vi "CODCr插入数据.vi"(0 "database":string, 1 "data":T3 {"单位" items=["ug/L", "mg/L", "ppm", "mg/m3", "cm", "ppb", "ug/m3", "%", "nmol/mol", "umol/mol", "MPN/L", "MPN/100ml", "ng/m3", "NTU", "无量纲", "ms/cm", "us/cm"]}, 5 "table":string, 7 "测量模式":T2(ring)=enum."水样测试", 9 "数据类型":enum16{"N", "M"}(ring)=enum."M", 11 "error in (no error)":errorcluster) -> (15 "error out":errorcluster)   [LabVIEW 2016, in "CODCr库.lvlib"]
uses:
  <vilib>/Utility/sysdir.llb/System Directory Type.ctl
  <vilib>/Utility/error.llb/DialogType.ctl
  <vilib>/addons/database/Auxilliary.llb/DB Tools Column Info.ctl
  <vilib>/addons/database/Auxilliary.llb/DB Tools DataTypes.ctl
  <vilib>/addons/database/Connection.llb/DB Tools Open Connec (String).vi
  <vilib>/addons/database/Connection.llb/Conn Execute.vi
  <vilib>/addons/database/Recordset.llb/Rec Destroy - Connection.vi
  <vilib>/addons/database/Recordset.llb/Rec Fetch Recordset Data (R).vi
  <vilib>/addons/database/NI_Database_API.lvlib
  WxMessage/wxpusher.lvlib
panel:
  out "data修正输出":T1
  out "data输出":T1
  out "为空？":bool
  out "recordset data":variant[][](array[variant])
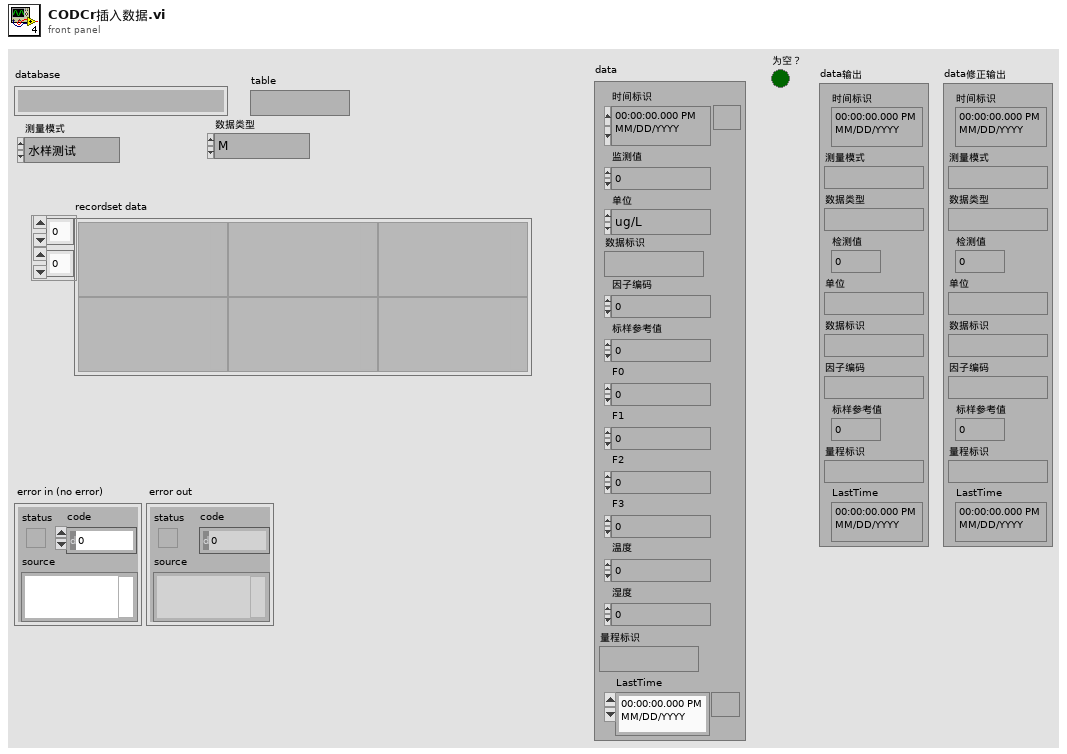
[diagram p1: front panel]
types:
  T1 = cluster{"时间标识":timestamp, "测量模式":string, "数据类型":string, "检测值":sgl, "单位":string, "数据标识":string, "因子编码":string, "标样参考值":sgl, "量程标识":string, "LastTime":timestamp}
  T2 = enum16{"空闲", "水样测试", "标样核查", "零点核查", "跨度核查", "空白测试", "平行样测试", "加标回收", "空白校准", "标样校准", "初始化（清洗）"}
  T3 = cluster{"时间标识":timestamp, "监测值":sgl, "单位":u16, "数据标识":string, "因子编码":u32, "标样参考值":sgl, "F0":sgl, "F1":sgl, "F2":sgl, "F3":sgl, "温度":sgl, "湿度":sgl, "量程标识":string, "LastTime":timestamp}
  T4 = typedef "DialogType.ctl" = u16
  T5 = typedef "System Directory Type.ctl" = i32
  T6 = typedef "NI_Database_API.lvlib/Conn ObjectReference.ctl" = refnum<k1>
  T7 = typedef "NI_Database_API.lvlib/Rec ObjectReference.ctl" = refnum<k1>
  T8 = typedef "NI_Database_API.lvlib/DB Tools Column Info.ctl" = cluster{"column name":string, "data type":T9, "size":i32, "allow null?":bool}
  T9 = typedef "NI_Database_API.lvlib/DB Tools DataTypes.ctl" = enum16{"String", "Long (I32)", "Single (SGL)", "Double (DBL)", "Date/Time", "Binary"}
  T10 = cluster{"测量量程":dbl, "测量精度":dbl, "测量间隔":dbl, "消解温度":dbl, "消解时长":dbl, "空白校准时间":timestamp, "曲线截距":dbl, "曲线斜率":dbl, "测量检出限":dbl, "测量信号值":dbl, "线性相关系数":dbl, "二次多项式系数":dbl, "标样校准时间":timestamp, "稀释倍数":dbl, "三项式系数":dbl, "空白标定系数":dbl, "量程系数":dbl, "F0/ORPA":dbl, "F1/ORPB":dbl, "F2/ORPK":dbl, "F3":dbl, "F4":dbl, "F5":dbl, "F6":dbl, "F7":dbl, "X0/滴定数":dbl, "量程":dbl}
  T11 = cluster{"切换阈值":dbl, "稳定系数":dbl, "变异系数":dbl, "enable":bool, "init":bool}
  T12 = cluster{"数值输出":dbl, "均值":dbl, "变异系数":dbl, "数据波动百分比":dbl, "随机数flag":bool}
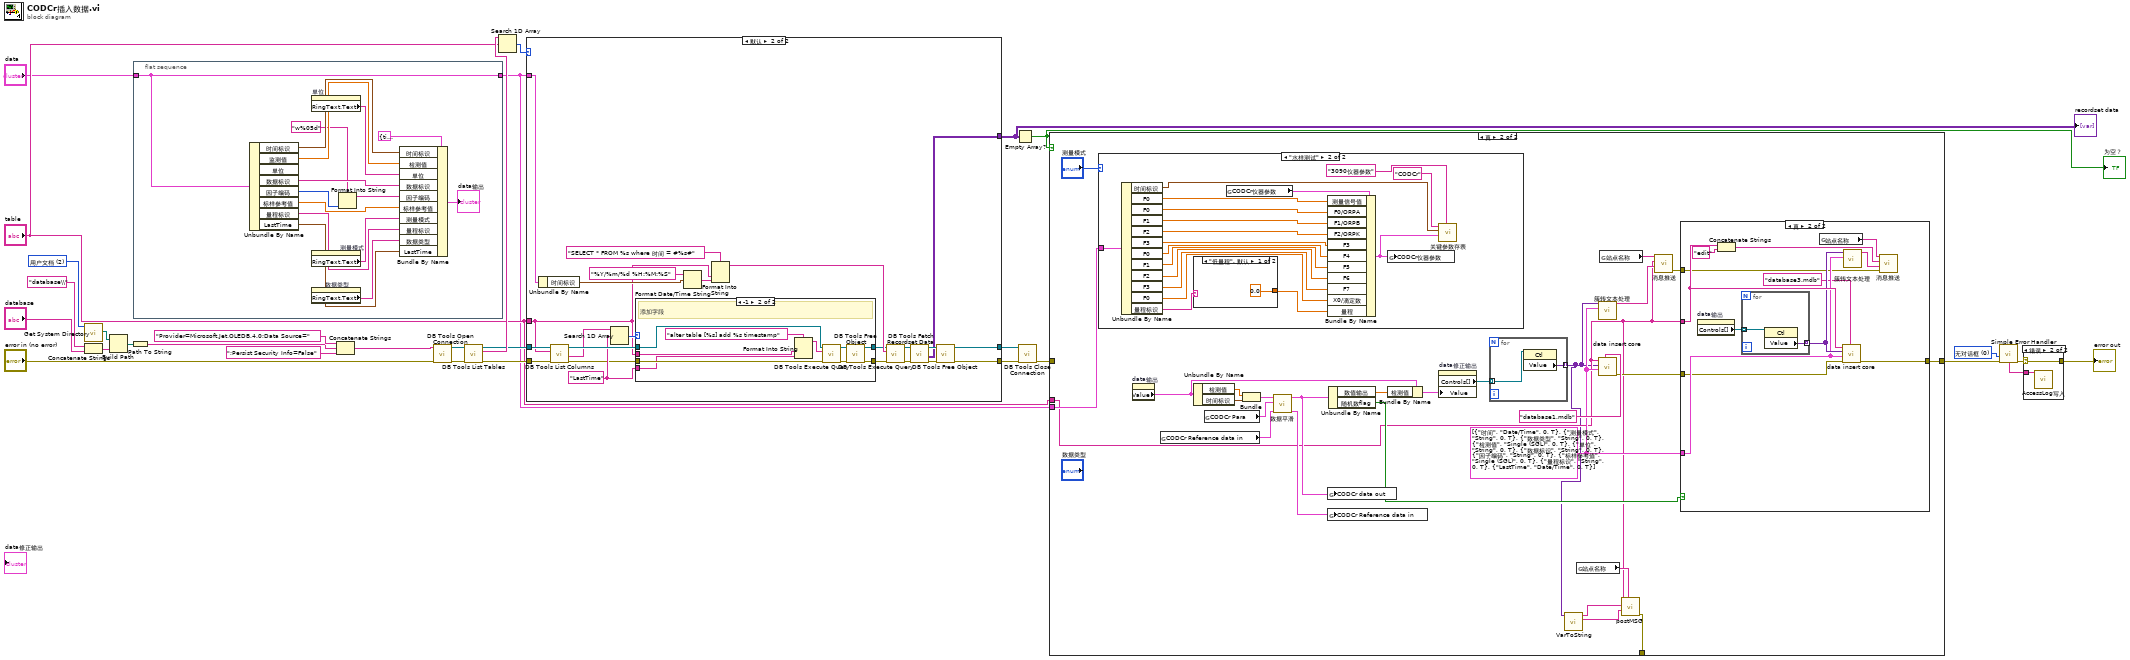
[diagram p0: block diagram]
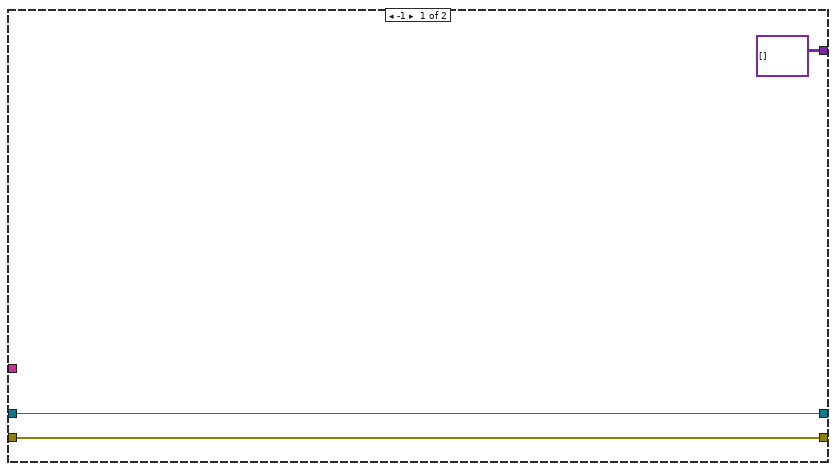
[diagram p3: hidden frame]
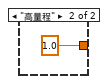
[diagram p8: hidden frame]
diagram:
  w11 = T4 0 items=["无对话框", "确定信息", "继续或停止信息", "确定信息＋警告", "继续/停止+警告"] ("type of dialog (OK msg:1)")
  w29 = T5 2 items=["用户目录"=0, "用户桌面"=1, "用户文档"=2, "用户应用程序数据"=3, "用户设置"=4, "用户临时目录"=5, "公共文档"=6, "公共应用程序数据"=7, "公共设置"=8, "公共缓存"=13, "系统核心库"=9, "系统安装库"=10, "应用程序文件"=11, "启动盘根目录"=12] ("system directory type")
  n1 = call <vilib>:"Get System Directory.vi"("system directory type"=w29) -> ("system directory"=w27:path)  [unwired: 10 in]
  n2 = Concatenate Strings("database\\" ("condition"), "database") -> (w21:string)
  n3 = Build Path(base path=w27, name or relative path=w21) -> (appended path=w26:path)
  n4 = Path To String(path=w26) -> (string=w25:string)
  n5 = flat-sequence {
    tunnel: "data" -> [w31]
    tunnel: [w31] -> w3
    frame #0 {
      n6 = Unbundle By Name(w31) -> ("时间标识"=w44:timestamp, "监测值"=w43:sgl, "数据标识"=w41:string, "因子编码"=w39:u32, "标样参考值"=w37:sgl, "量程标识"=w35:string, "LastTime"=w33:timestamp)  [unwired: 1 out]
      n7 = property on="单位" class="Ring (严格)"() -> ("RingText.Text"=w42:string)  [unwired: 2 in, 2 out]
      n8 = property on="测量模式" class="Enum (严格)"() -> ("RingText.Text"=w36:string)  [unwired: 2 in, 2 out]
      n9 = property on="数据类型" class="Enum (严格)"() -> ("RingText.Text"=w34:string)  [unwired: 2 in, 2 out]
      n10 = Format Into String(format string="w%05d" ("格式字符串"), w39) -> (resulting string=w38:string)  [unwired: 2 in, 1 out]
      n11 = Bundle By Name(cluster=T1 {"时间标识"=timestamp(0 s since 1904-01-01), "测量模式"="", "数据类型"="", "检测值"=0.0, "单位"="", "数据标识"="", "因子编码"="", "标样参考值"=0.0, "量程标识"="", "LastTime"=timestamp(0 s since 1904-01-01)} ("data输出"), "时间标识"=w44, "检测值"=w43, "单位"=w42, "数据标识"=w41, "因子编码"=w38, "标样参考值"=w37, "测量模式"=w36, "量程标识"=w35, "数据类型"=w34, "LastTime"=w33) -> (→"data输出":T1)
    }
  }
  n12 = Concatenate Strings("Provider=Microsoft.Jet.OLEDB.4.0;Data Source=" ("condition"), w25, ";Persist Security Info=False" ("condition")) -> (w23:string)
  n13 = call-poly <vilib>:"DB Tools Open Connection.vi"("error in (no error)"="error in (no error)", "connection information"=w23) -> ("error out"=w19:errorcluster, "connection reference"=w20:T6)  [unwired: 6 in]
  n14 = call <vilib>:"DB Tools List Tables.vi"("error in (no error)"=w19, "connection reference"=w20) -> ("error out"=w14:errorcluster, "tables"=w18:string[], "connection reference out"=w15:T6)  [unwired: 3 in]
  n15 = Search 1D Array(1D array=w18, element="table") -> (index of element=w13:i32)  [unwired: 1 in]
  n16 = case shown="默认" w13 {
    tunnel: [variant[][] [] ("recordset data") w67] -> w12
    tunnel: [w48 w66] -> w7
    tunnel: [w47 w65] -> w6
    tunnel: w15 -> [w48 w52]
    tunnel: w14 -> [w47 w51]
    tunnel: "table" -> [_ w50]
    tunnel: w3 -> [_ w60]
    frame -1 {
    }
    frame Default {
      w58 = "LastTime" ("元素")
      n17 = Unbundle By Name(w60) -> ("时间标识"=w63:timestamp)
      n18 = call <vilib>:"DB Tools List Columns.vi"("error in (no error)"=w51, "table"=w50, "connection reference"=w52) -> ("error out"=w56:errorcluster, "columns"=w57:string[], "connection reference out"=w59:T6)  [unwired: 1 in, 1 out]
      n19 = Search 1D Array(1D array=w57, element=w58) -> (index of element=w55:i32)  [unwired: 1 in]
      n20 = case shown="-1" w55 {
        tunnel: w59 -> [w73 w81]
        tunnel: w56 -> [w72 w80]
        tunnel: w58 -> [_ w78]
        tunnel: [w73 w76] -> w54
        tunnel: [w72 w75] -> w53
        tunnel: w50 -> [_ w74]
        frame 0, Default {
        }
        frame -1 {
          # "添加字段"
          n21 = Format Into String(format string="alter table [%s] add %s timestamp", w74, w78) -> (resulting string=w77:string)  [unwired: 2 in, 1 out]
          n22 = call-poly <vilib>:"DB Tools Execute Query.vi"("error in (no error)"=w80, "SQL query"=w77, "connection reference"=w81) -> ("error out"=w82:errorcluster, "recordset reference"=w83:T7)  [unwired: 5 in]
          n23 = call-poly <vilib>:"DB Tools Free Object.vi"("error in (no error)"=w82, "recordset reference"=w83) -> ("error out"=w75:errorcluster, "connection reference"=w76:T6)  [unwired: 8 in]
        }
      }
      n24 = Format Date/Time String(time format string (%c)="%Y/%m/%d %H:%M:%S" ("时间格式字符串(%c)"), seconds (now)=w63) -> (date/time string=w61:string)  [unwired: 1 in]
      n25 = Format Into String(format string="SELECT * FROM %s where 时间 = #%s#" ("格式字符串"), w50, w61) -> (resulting string=w64:string)  [unwired: 2 in, 1 out]
      n26 = call-poly <vilib>:"DB Tools Execute Query.vi"("error in (no error)"=w53, "SQL query"=w64, "connection reference"=w54) -> ("error out"=w68:errorcluster, "recordset reference"=w71:T7)  [unwired: 5 in]
      n27 = call-poly <vilib>:"DB Tools Fetch Recordset Data.vi"("error in (no error)"=w68, "recordset reference"=w71) -> ("error out"=w69:errorcluster, "recordset data"=w67:variant[][], "recordset reference out"=w70:T7)  [unwired: 3 in]
      n28 = call-poly <vilib>:"DB Tools Free Object.vi"("error in (no error)"=w69, "recordset reference"=w70) -> ("error out"=w65:errorcluster, "connection reference"=w66:T6)  [unwired: 8 in]
    }
  }
  "recordset data" <- w12
  n29 = Empty Array?(array=w12) -> (empty?=w16:bool)
  "为空？" <- w16
  n30 = call <vilib>:"DB Tools Close Connection.vi"("error in (no error)"=w6, "connection reference"=w7) -> ("error out"=w5:errorcluster)  [unwired: 5 in]
  n31 = case shown="真" w16 {
    tunnel: "table" -> [_ w89]
    tunnel: w3 -> [_ w111]
    tunnel: w5 -> [w84 _]
    tunnel: [w84 w91] -> w1
    tunnel: [_ w85] -> _
    frame False {
    }
    frame True {
      w93 = T8[] [{"column name"="时间", "data type"=enum."Date/Time", "size"=0, "allow null?"=TRUE}, {"column name"="测量模式", "data type"=enum."String", "size"=0, "allow null?"=TRUE}, {"column name"="数据类型", "data type"=enum."String", "size"=0, "allow null?"=TRUE}, {"column name"="检测值", "data type"=enum."Single (SGL)", "size"=0, "allow null?"=TRUE}, {"column name"="单位", "data type"=enum."String", "size"=0, "allow null?"=TRUE}, {"column name"="数据标识", "data type"=enum."String", "size"=0, "allow null?"=TRUE}, {"column name"="因子编码", "data type"=enum."String", "size"=0, "allow null?"=TRUE}, {"column name"="标样参考值", "data type"=enum."Single (SGL)", "size"=0, "allow null?"=TRUE}, {"column name"="量程标识", "data type"=enum."String", "size"=0, "allow null?"=TRUE}, {"column name"="LastTime", "data type"=enum."Date/Time", "size"=0, "allow null?"=TRUE}] ("column information")
      n32 = case shown="\"水样测试\"" "测量模式" {
        tunnel: w111 -> [_ w129]
        frame "空闲", Default {
        }
        frame "水样测试" {
          n33 = Unbundle By Name(w129) -> ("时间标识"=w145:timestamp, "F0"=w144:sgl, "F0"=w132:sgl, "F1"=w133:sgl, "F2"=w134:sgl, "F3"=w135:sgl, "F0"=w136:sgl, "F1"=w137:sgl, "F2"=w138:sgl, "F3"=w139:sgl, "F0"=w140:sgl, "量程标识"=w142:string)
          n34 = case shown="\"低量程\", 默认" w142 {
            tunnel: [0.0 ("量程") 1.0 ("量程")] -> w141
            frame "低量程", Default {
            }
            frame "高量程" {
            }
          }
          n35 = global read "CODcr全局变量.vi" "CODCr仪器参数"() -> (w131:T10)
          n36 = Bundle By Name(cluster=w131, "测量信号值"=w144, "F0/ORPA"=w132, "F1/ORPB"=w133, "F2/ORPK"=w134, "F3"=w135, "F4"=w136, "F5"=w137, "F6"=w138, "F7"=w139, "X0/滴定数"=w140, "量程"=w141) -> (w130:T10)
          n37 = global write "CODcr全局变量.vi" "CODCr仪器参数"(w130) -> ()
          n38 = call "关键参数存表.vi"("table"="3090仪器参数", "仪器参数"=w130, "datatime"=w145, "仪器名称"="CODCr") -> ()  [unwired: 7 in, 1 out]
        }
      }
      n39 = property on="data输出" class="Clust (严格)"() -> ("Value"=w101:T1)  [unwired: 2 in, 2 out]
      n40 = global read "仿真全局变量.vi" "CODCr Reference data in"() -> (w105:cluster{"参考数值":dbl[], "参考数值时间戳":timestamp[]})
      n41 = Unbundle By Name(w101) -> ("检测值"=w108:sgl, "时间标识"=w107:timestamp)
      n42 = global read "仿真全局变量.vi" "CODCr Para"() -> (w104:T11)
      n43 = Bundle("检测值"=w108, "时间标识"=w107) -> (w106:cluster{"检测值":sgl, "时间标识":timestamp})  [unwired: 1 in]
      n44 = call "数据平滑.vi"("Reference data in"=w105, "Para"=w104, "data in"=w106) -> ("Reference data out"=w103:cluster{"参考数值":dbl[], "参考数值时间戳":timestamp[]}, "data out"=w100:T12)  [unwired: 7 in]
      n45 = global write "仿真全局变量.vi" "CODCr data out"(w100) -> ()
      n46 = global write "仿真全局变量.vi" "CODCr Reference data in"(w103) -> ()
      n47 = Unbundle By Name(w100) -> ("数值输出"=w99:dbl, "随机数flag"=w95:bool)
      n48 = Bundle By Name(cluster=w101, "检测值"=w99) -> (w98:T1)
      n49 = property on="data修正输出" class="Clust (严格)"("Value"=w98) -> ("Controls[]"=w102:refnum<vi>[])  [unwired: 2 in, 2 out]
      n50 = for {
        tunnel: w102 -> [w128] mode=indexing
        tunnel: [w127] -> w86 mode=indexing
        n51 = property class="Ctl"(reference=w128) -> ("Value"=w127:variant)  [unwired: 1 in, 2 out]
      }
      n52 = call "VarToString.vi"("数组"=w86) -> ("data"=w87:string[], "columns"=w88:string[])  [unwired: 9 in]
      n53 = global read "系统设置全局变量.vi" "站点名称"() -> (w90:string)
      n54 = call "簇转文本处理.vi"("column information"=w93, "data"=w86) -> ("output"=w97:string)  [unwired: 9 in]
      n55 = call "data insert core.vi"("database"="database1.mdb", "column information"=w93, "data"=w86, "table"=w89) -> ("error out"=w92:errorcluster)  [unwired: 7 in]
      n56 = global read "系统设置全局变量.vi" "站点名称"() -> (w96:string)
      n57 = call "postMSG.vi"("station"=w90, "data"=w87, "columns"=w88, "table"=w89) -> ("error out"=w85:errorcluster)  [unwired: 7 in]
      n58 = call "消息推送.vi"("数据内容"=w97, "参数"=w89, "站点"=w96) -> ("error out"=w94:errorcluster)  [unwired: 8 in]
      n59 = case shown="真" w95 {
        tunnel: w94 -> [_ w114]
        tunnel: w89 -> [_ w119]
        tunnel: w93 -> [_ w117]
        tunnel: w92 -> [w112 w116]
        tunnel: [w112 w115] -> w91
        frame False {
        }
        frame True {
          n60 = property on="data输出" class="Clust (严格)"() -> ("Controls[]"=w120:refnum<vi>[])  [unwired: 2 in, 2 out]
          n61 = Concatenate Strings(w119, "edit" ("字符串")) -> (w121:string)
          n62 = for {
            tunnel: w120 -> [w126] mode=indexing
            tunnel: [w125] -> w118 mode=indexing
            n63 = property class="Ctl"(reference=w126) -> ("Value"=w125:variant)  [unwired: 1 in, 2 out]
          }
          n64 = global read "系统设置全局变量.vi" "站点名称"() -> (w124:string)
          n65 = call "data insert core.vi"("database"="database3.mdb", "error in (no error)"=w116, "column information"=w117, "data"=w118, "table"=w119) -> ("error out"=w115:errorcluster)  [unwired: 6 in]
          n66 = call "簇转文本处理.vi"("column information"=w117, "data"=w118) -> ("output"=w123:string)  [unwired: 9 in]
          n67 = call "消息推送.vi"("error in (no error)"=w114, "数据内容"=w123, "参数"=w121, "站点"=w124) -> ()  [unwired: 7 in, 1 out]
        }
      }
    }
  }
  n68 = call <vilib>:"Simple Error Handler.vi"("type of dialog (OK msg:1)"=w11, "error in (no error)"=w1) -> ("error out"=w10:errorcluster, "message"=w9:string)  [unwired: 3 in, 3 out]
  n69 = case shown="错误" w10 {
    selector: w10 -> [w149 w150]
    tunnel: w9 -> [_ w151]
    tunnel: [w149 w150] -> w2
    frame No Error {
    }
    frame Error {
      n70 = call "AccessLog写入.vi"("Log"=w151) -> ()  [unwired: 11 in]
    }
  }
  "error out" <- w2
